vi "Clear.vi"(8 "error in (no error)":errorcluster, 11 "Execution UI In":refnum<class "Execution UI.lvclass">) -> (0 "error out":errorcluster)   [LabVIEW 2020, in "Execution UI.lvclass"]
uses:
  Execution UI.lvclass
  Execution UI.lvclass/Execution UI.ctl
  Result Model by Reference/Result Model by Reference.lvclass
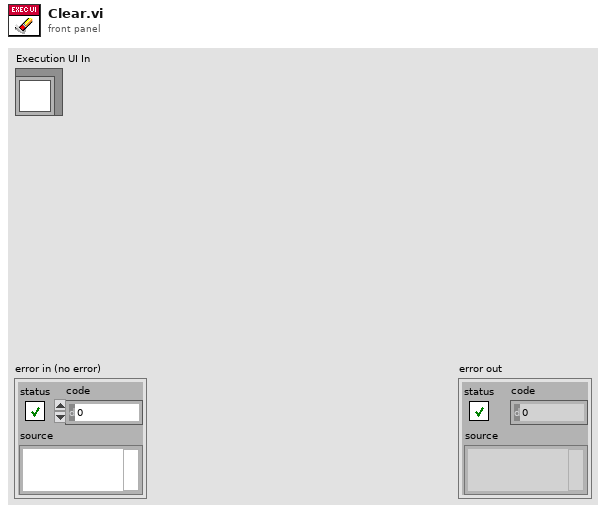
[diagram p1: front panel]
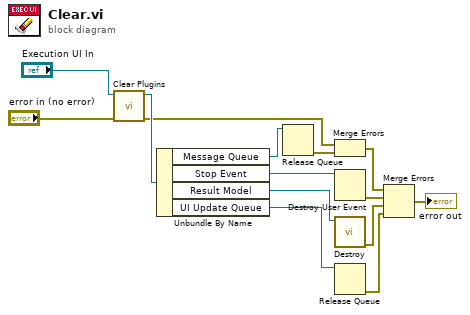
[diagram p0: block diagram]
diagram:
  n1 = call "Clear Plugins.vi"("error in (no error)"="error in (no error)", "Execution UI in"="Execution UI In") -> ("error out"=w4:errorcluster, "Execution UI out"=w5:refnum<class "Execution UI.lvclass">)  [unwired: 8 in]
  n2 = Unbundle By Name(w5) -> ("Message Queue"=w1:refnum<queue>, "Stop Event"=w12:refnum<user-event>, "Result Model"=w10:refnum<class "Result Model by Reference.lvclass">, "UI Update Queue"=w8:refnum<queue>)
  n3 = Release Queue(queue=w1) -> (error out=w2:errorcluster)  [unwired: 2 in, 2 out]
  n4 = Merge Errors(w4, w2) -> (w3:errorcluster)
  n5 = Destroy User Event(user event=w12) -> (error out=w11:errorcluster)  [unwired: 1 in]
  n6 = call "Destroy.vi"("Result Model in"=w10) -> ("error out"=w9:errorcluster)  [unwired: 10 in]
  n7 = Release Queue(queue=w8) -> (error out=w7:errorcluster)  [unwired: 2 in, 2 out]
  n8 = Merge Errors(w3, w11, w9, w7) -> (→"error out":errorcluster)
